vi "CoreState_Init.vi"(8 "error in (no error)":errorcluster, 11 "Sim DiscreteIO in":refnum<class "Sim DiscreteIO.lvclass">) -> (0 "error out":errorcluster, 3 "Sim DiscreteIO out":refnum<class "Sim DiscreteIO.lvclass">)   [LabVIEW 2021, in "Sim DiscreteIO.lvclass"]
uses:
  Sim DiscreteIO.lvclass
  TypeDefs/DVR.ctl
  TypeDefs/_PARMS.ctl
  Sim DiscreteIO.lvclass/Sim DiscreteIO.ctl
  <userlib>/S2 Labs/Module Framework/Modules/Base/Module.lvclass
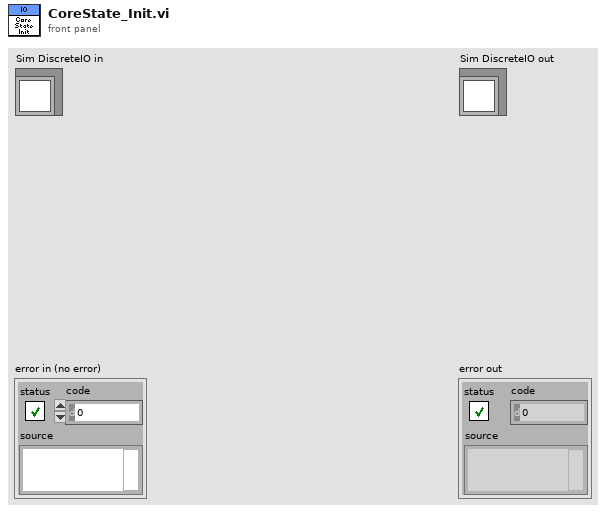
[diagram p1: front panel]
types:
  T1 = typedef "Sim DiscreteIO.lvclass/DVR.ctl" = cluster{"ch_labels":string[], "_PARMS":T2, "Initialized?":bool, "occurrence":refnum<k4>}
  T2 = typedef "Sim DiscreteIO.lvclass/_PARMS.ctl" = cluster{"ch_units":string[], "ch_alias":string[]}
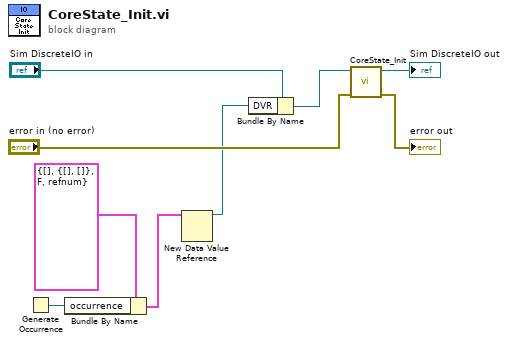
[diagram p0: block diagram]
diagram:
  n1 = Generate Occurrence() -> (w1:refnum<k4>)
  n2 = Bundle By Name(cluster=T1 {"ch_labels"=[], "_PARMS"={"ch_units"=[], "ch_alias"=[]}, "Initialized?"=FALSE, "occurrence"=refnum} ("DVR"), "occurrence"=w1) -> (w2:T1)
  n3 = New Data Value Reference(data value=w2) -> (data value reference=w4:refnum<data-value>)  [unwired: 1 in, 1 out]
  n4 = Bundle By Name(cluster="Sim DiscreteIO in", "DVR"=w4) -> (w5:refnum<class "Sim DiscreteIO.lvclass">)
  n5 = call-parent "CoreState_Init.vi"("error in (no error)"="error in (no error)", "Module in"=w5) -> ("error out"=→"error out":errorcluster, "Module out"=→"Sim DiscreteIO out":refnum<class "Sim DiscreteIO.lvclass">)  [unwired: 8 in]
